vi "testdrive.vi"() -> ()   [LabVIEW 2012]
uses:
  <vilib>/Rock Robotics/SystemInterfaces/DIO/FPGA_DIOPWMChannel.ctl
  <vilib>/Rock Robotics/WPI/Joystick/WPI_JoystickDeviceEnum.ctl
  <vilib>/Rock Robotics/WPI/Joystick/WPI_JoystickAxis.ctl
  <vilib>/Rock Robotics/WPI/RobotDrive/WPI_RobotDriveOpen2MotorWithTalon.vi
panel:
  in  "stop":bool
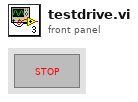
[diagram p1: front panel]
types:
  T1 = typedef "WPI_JoystickDeviceEnum.ctl" = enum16{"USB 1", "USB 2", "USB 3", "USB 4", "Kinect 1", "Kinect 2"}
  T2 = typedef "FPGA_DIOPWMChannel.ctl" = enum8{"PWM 1", "PWM 2", "PWM 3", "PWM 4", "PWM 5", "PWM 6", "PWM 7", "PWM 8", "PWM 9", "PWM 10", "Invalid"}
  T3 = typedef "WPI_JoystickDevRef.ctl" = cluster{"Device":T1}
  T4 = typedef "WPI_RobotDriveDevRef.ctl" = cluster{"DevStatus":errorcluster, "Motors[]":T5[], "Square Inputs":bool, "Max Output":dbl, "Isochronous":bool}
  T5 = typedef "WPI_MotorControlDeviceRef.ctl" = cluster{"DeviceStatus":errorcluster, "Type":enum16{"PWM", "CAN"}, "PWM":cluster{"Digital Module":T6, "PWM Channel":T2, "DeadBand":T7}, "CAN":cluster{"Device Number":u8, "Control Mode":T8, "Semaphore":T9, "Max Vout":dbl}, "Invert":bool, "TransformRef":T10, "InvTransformRef":T10}
  T6 = typedef "FPGA_TypedefDigitalModule.ctl" = enum16{"Digital Module 1", "Digital Module 2"}
  T7 = typedef "WPI_PWMDeadband.ctl" = cluster{"Name":string, "maxPositivePwm":i32, "minPositivePwm":i32, "centerPwm":i32, "maxNegativePwm":i32, "minNegativePwm":i32, "angularRange":u16}
  T8 = typedef "WPI_CANJaguar_ControlMode.ctl" = enum8{"Percent VBus", "Current", "Speed", "Position", "Voltage"}
  T9 = typedef "Semaphore RefNum" = refnum<k1>
  T10 = typedef "WPI_PWMTransform_ConPane.ctl" = refnum<vi>
  T11 = typedef "WPI_JoystickAxis.ctl" = enum16{"Axis 1", "Axis 2", "Axis 3", "Axis 4", "Axis 5", "Axis 6"}
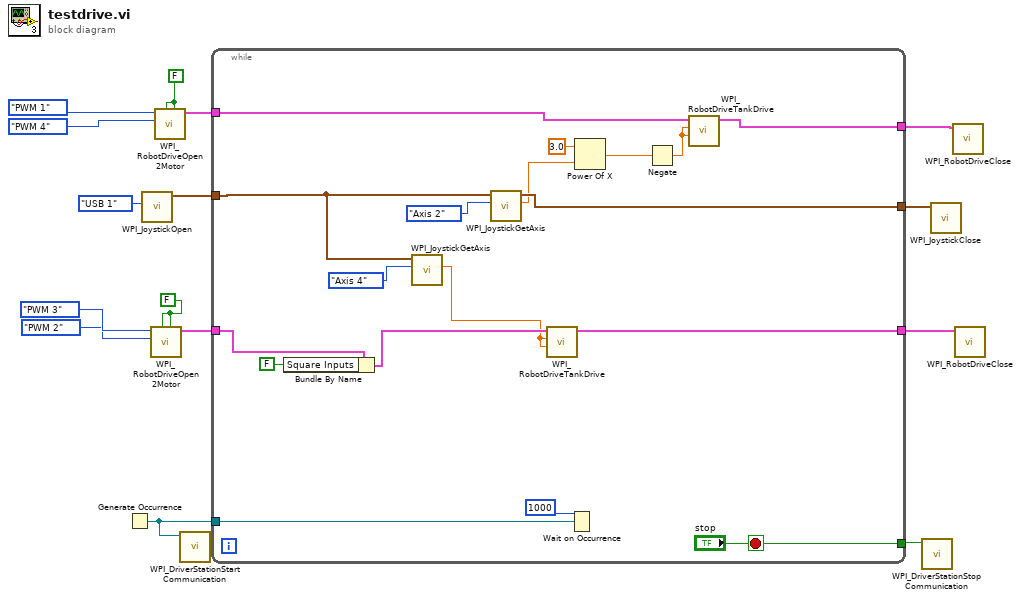
[diagram p0: block diagram]
diagram:
  w2 = FALSE ("Right Motor Inverted")
  w3 = FALSE ("Right Motor Inverted")
  n1 = Generate Occurrence() -> (w15:refnum<k4>)
  n2 = call <vilib>:"WPI_JoystickOpen.vi"("JoystickDevice"=WPI_JoystickDeviceEnum."USB 1") -> ("JoystickDevRef"=w7:T3)  [unwired: 10 in]
  n3 = call-poly <vilib>:"WPI_RobotDriveOpen2Motor.vi"("LB Inverted"=w2, "LF Inverted"=w2, "Left Motors"=FPGA_DIOPWMChannel."PWM 2" ("Right Motor"), "Right Motors"=FPGA_DIOPWMChannel."PWM 3" ("Left Motor")) -> ("RobotDriveDevRef"=w8:T4)  [unwired: 6 in, 1 out]
  n4 = call-poly <vilib>:"WPI_RobotDriveOpen2Motor.vi"("LB Inverted"=w3, "LF Inverted"=w3, "Left Motors"=FPGA_DIOPWMChannel."PWM 4" ("Right Motor"), "Right Motors"=FPGA_DIOPWMChannel."PWM 1" ("Left Motor")) -> ("RobotDriveDevRef"=w9:T4)  [unwired: 6 in, 1 out]
  n5 = call <vilib>:"WPI_DriverStationStart Communication.vi"("occurrence"=w15) -> ()  [unwired: 11 out]
  n6 = while {
    tunnel: w15 -> [w33]
    tunnel: ["stop"] -> w14
    tunnel: w9 -> [w21]
    tunnel: w8 -> [w25]
    tunnel: w7 -> [w26]
    tunnel: [w30] -> w6
    tunnel: [w28] -> w5
    tunnel: [w20] -> w4
    stop <- "stop" stop-if-true
    n7 = Bundle By Name(cluster=w25, "Square Inputs"=FALSE) -> (w23:T4)
    n8 = call <vilib>:"WPI_JoystickGetAxis.vi"("Axis"=WPI_JoystickAxis."Axis 4", "JoystickDevRef"=w26) -> ("Value"=w22:dbl)  [unwired: 8 in, 1 out]
    n9 = call <vilib>:"WPI_JoystickGetAxis.vi"("Axis"=WPI_JoystickAxis."Axis 2", "JoystickDevRef"=w26) -> ("Value"=w19:dbl, "JoystickDevRef"=w20:T3)  [unwired: 8 in]
    n10 = call <vilib>:"WPI_RobotDriveTankDrive.vi"("Right axis value"=w22, "Left axis value"=w22, "RobotDriveDevRef"=w23) -> ("RobotDriveDevRef"=w28:T4)  [unwired: 6 in, 2 out]
    n11 = Wait on Occurrence(2:w33, 3:1000 ("ms timeout (-1)")) -> ()  [unwired: 2 out]
    n12 = Power Of X(1:w19, 2:3.0 ("y")) -> (0:w16:dbl)
    n13 = Negate(x=w16) -> (-x=w17:dbl)
    n14 = call <vilib>:"WPI_RobotDriveTankDrive.vi"("Right axis value"=w17, "Left axis value"=w17, "RobotDriveDevRef"=w21) -> ("RobotDriveDevRef"=w30:T4)  [unwired: 6 in, 2 out]
  }
  n15 = call <vilib>:"WPI_DriverStationStop Communication.vi"("StopCommunication"=w14) -> ()  [unwired: 1 in, 10 out]
  n16 = call <vilib>:"WPI_JoystickClose.vi"("JoystickDevRef"=w4) -> ()  [unwired: 11 in]
  n17 = call <vilib>:"WPI_RobotDriveClose.vi"("RobotDriveDevRef"=w6) -> ()  [unwired: 10 in, 1 out]
  n18 = call <vilib>:"WPI_RobotDriveClose.vi"("RobotDriveDevRef"=w5) -> ()  [unwired: 10 in, 1 out]
